vi "Force_2.vi"() -> ()   [LabVIEW 2020]
uses:
  Support/Controls/Cmd_Mouse Popup.ctl
  Support/Controls/Cmd_Var Data IO.ctl
  Support/Controls/Clst_Initialize Input.ctl
  Support/Controls/Clst_Result inspec.ctl
  Support/Public/Polymorph/Data Class_2D Str.vi
  Variables/Global_Cal Info.vi
  Support/Public/Polymorph/Rmv Empt Arr_2D Str.vi
panel:
  in  "Result set 2":string[][][](array[string])
  in  "Measured_ADJ":string[][](table) caption="● 측정 데이터 (조정후)"
  out "std set":string[][](table) caption="○ 분동 세트"
  in  "Spec Default set":string[][][](array[string])
  in  "Result set":string[][][](array[string])
  in  "CMC set":string[][][](array[string])
  in  "Resolution":string[][][](array[string])
  in  "condition 변경":bool
  in  "Spec set":string[][][](array[string])
  in  "Condition set":string[][][](array[string])
  in  "삭제":bool
  in  "단 선택":T1(ring)
  in  "dut info":i32(listbox) caption="교정대상 기기 정보"
  in  "Measured":string[][](table) caption="● 측정 데이터"
  in  "초기화":bool
  in  "적용":bool
  in  "지시형태":string(combo)="Digital"
  in  "교정범위":string(combo)="20 ~ 90 %"
  in  "사용 기준기":string(combo)
  in  "측정점 수":u8=5
  in  "단위":string(combo)="N"
  in  "최대 용량":dbl=10.0
  out "교정 방향":string="압축"
  in  "Spec 변경":bool
  in  "Random":bool
  out "Spec":string[][](table)
  out "제목":string
  out "에러 출력":errorcluster
  in  "최소눈금":dbl=0.001
  in  "Condition":string[][](table) caption="○ 상대지시 오차 교정"
  out "Load?":bool
  # "※ 교정하중 값을 변경하고 변경 적용 버튼을 클릭 !!"
  # "1차 (0˚)"
  # "2차 (120˚)"
  # "3차 (240˚)"
  # "1차 (0˚)"
  # "2차 (120˚)"
  # "3차 (240˚)"
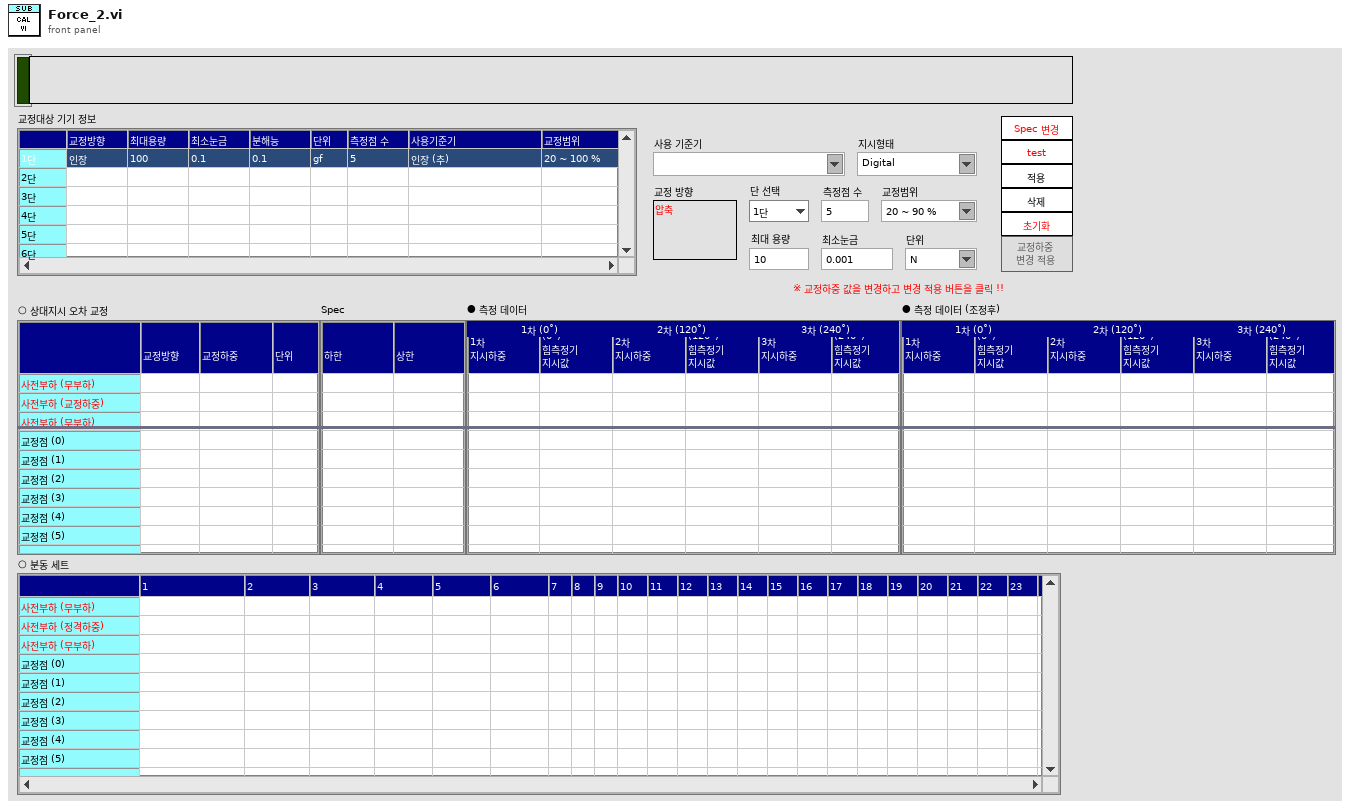
[diagram p1: front panel]
types:
  T1 = enum8{"1단", "2단", "3단", "4단", "5단", "6단", "7단", "8단", "9단", "10단"}
  T2 = typedef "Cmd_Mouse Popup.ctl" = enum16{"활성화", "메뉴선택"}
  T3 = typedef "Cmd_Var Data IO.ctl" = enum16{"Condition", "Condition Default", "Condition_Temp", "Resolution", "Resolution Default", "Resolution Old", "Spec", "Spec Default", "Spec Old", "Spec Temp", "Result", "Result2", "Result3", "Result_Temp", "Result_ADJ", "Result_ADJ2", "STD1", "STD2", "STD3", "STD4", "STD5", "STD Temp", "CMC", "CMC Default"}
  T4 = enum8{"Enabled", "Disabled", "Disabled and Grayed Out"}
  T5 = cluster{"Shift":bool, "Ctrl":bool, "Alt":bool, "Cmd":bool, "Opt":bool}
  T6 = typedef "Clst_Initialize Input.ctl" = cluster{"Initialize 1":cluster{"Condition":refnum<vi>[], "Spec":refnum<vi>[], "Measured":refnum<vi>[], "Resolution":refnum<vi>[], "Func_ext":string, "제목":refnum<vi>, "Measured_ADJ":refnum<vi>[]}, "Initialize 2":cluster{"문자열":refnum<vi>[], "콤보박스":refnum<vi>[], "링":refnum<vi>[], "열거형":refnum<vi>[], "테이블":refnum<vi>[], "여러열":refnum<vi>[], "디지털(DBL)":refnum<vi>[], "3D string":refnum<vi>[], "ctrl":refnum<vi>[], "boolean":refnum<vi>[]}}
  T7 = typedef "Clst_Result inspec.ctl" = cluster{"분해능":string, "문자열 1":string, "문자열 2":string, "숫자형 1":i32, "숫자형 2":i32, "숫자형 3":dbl, "문자배열 1D":string[], "문자배열 2D":string[][], "문자배열 3D":string[][][], "문자배열 4D":string[][][][], "불리언 1D":bool[]}
  T8 = cluster{"교정 방향":string, "최대 용량":dbl, "최소눈금":dbl, "지시형태":string, "단위":string, "측정점 수":u8, "사용 기준기":string, "사용 기준기 2":string, "단 선택":enum8{"1단", "2단", "3단", "4단", "5단", "6단", "7단", "8단", "9단", "10단"}, "ItemNames":string[][]}
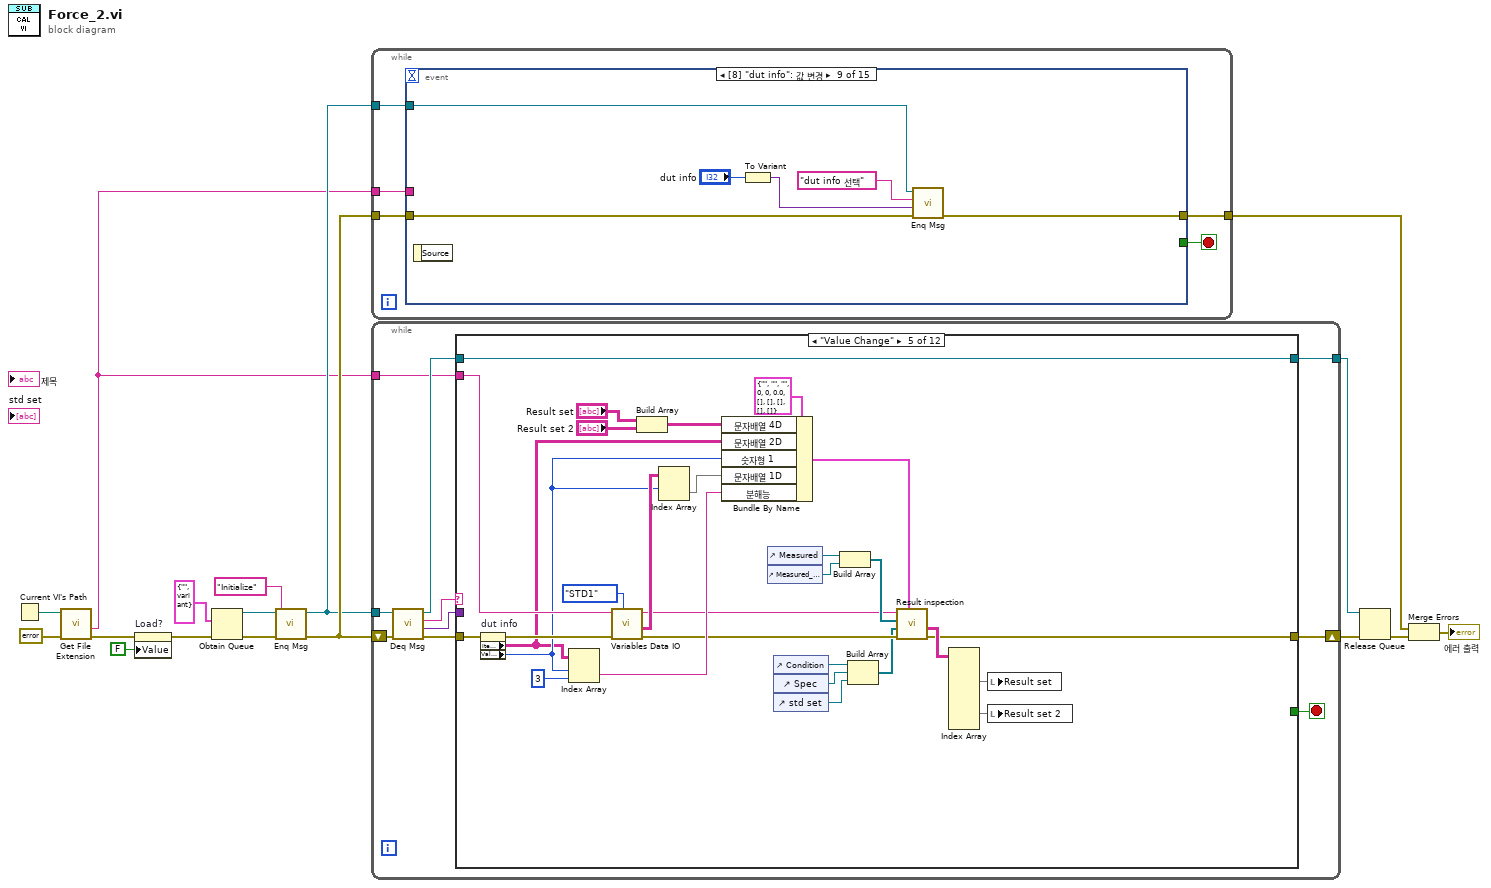
[diagram p0: block diagram]
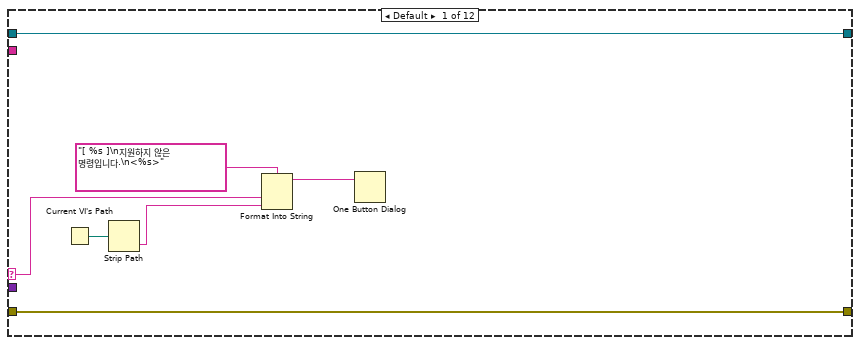
[diagram p2: hidden frame]
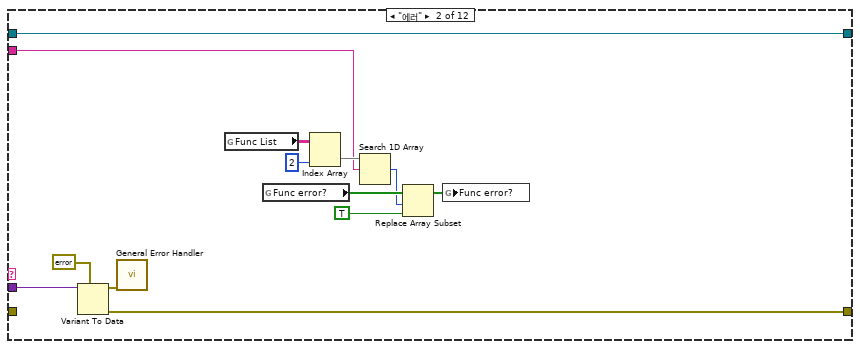
[diagram p3: hidden frame]
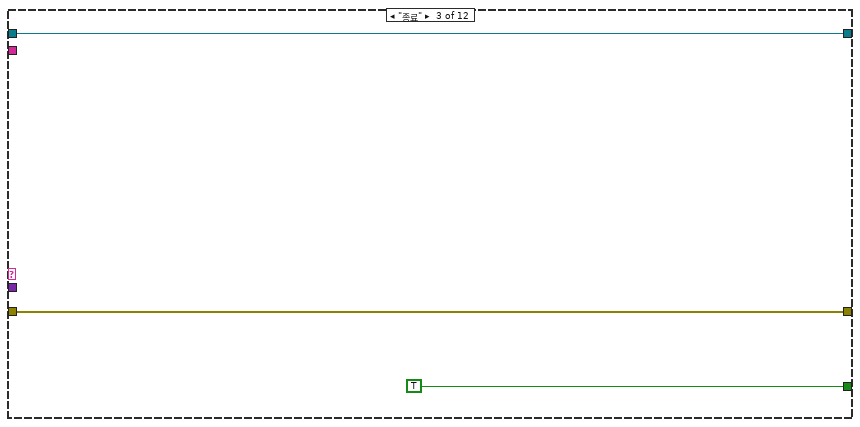
[diagram p4: hidden frame]
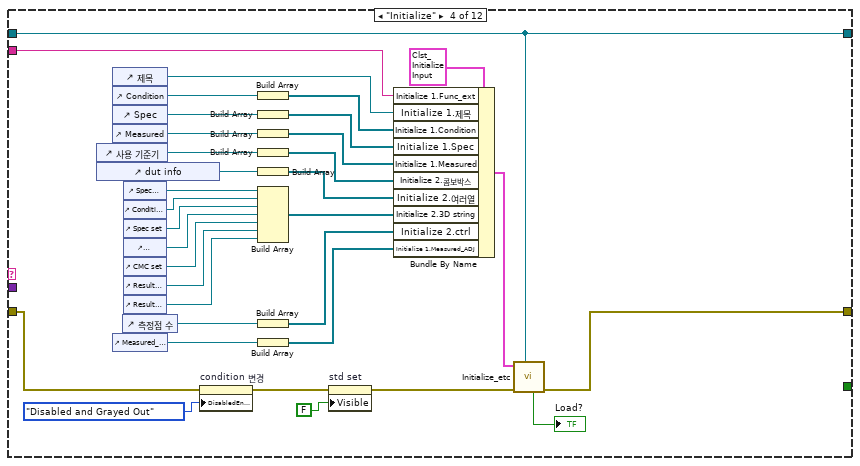
[diagram p5: hidden frame]
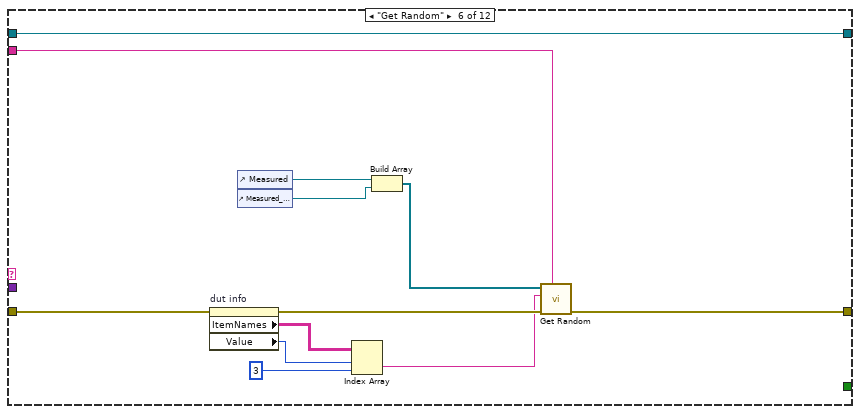
[diagram p6: hidden frame]
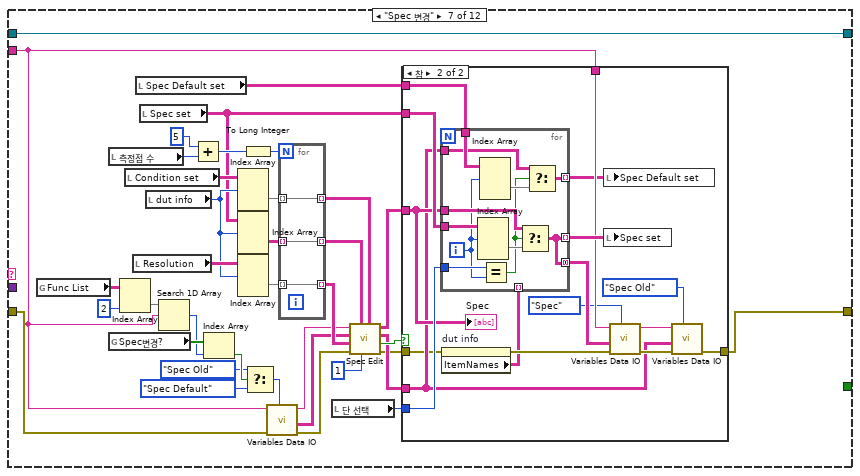
[diagram p7: hidden frame]
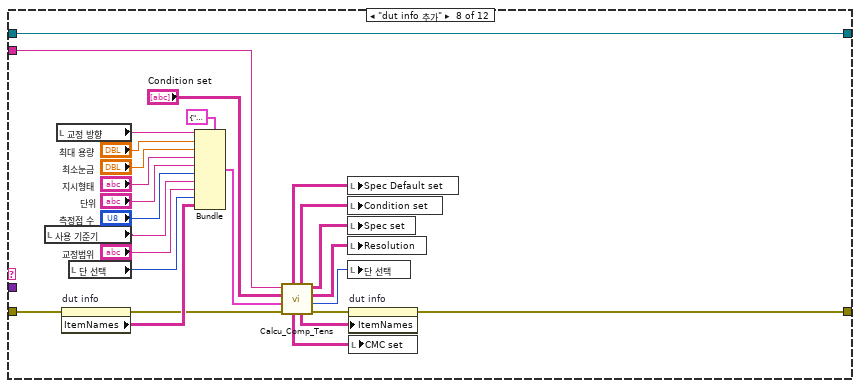
[diagram p9: hidden frame]
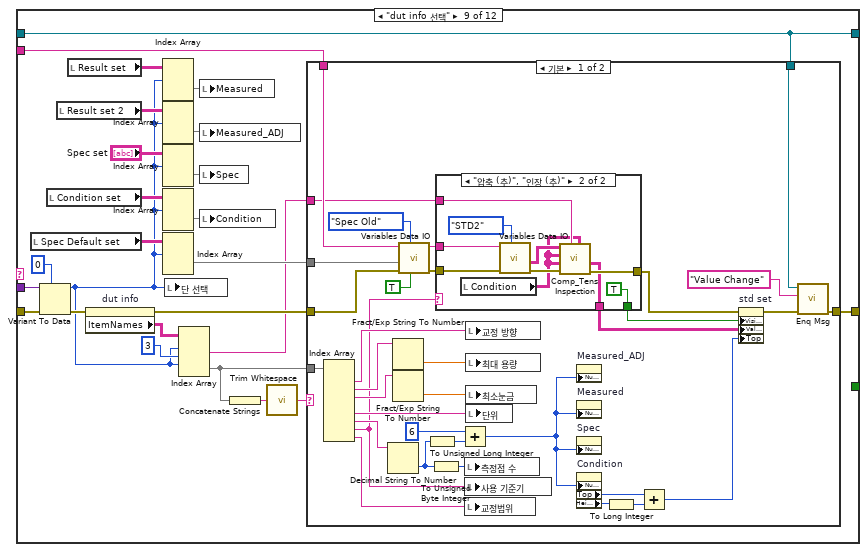
[diagram p10: hidden frame]
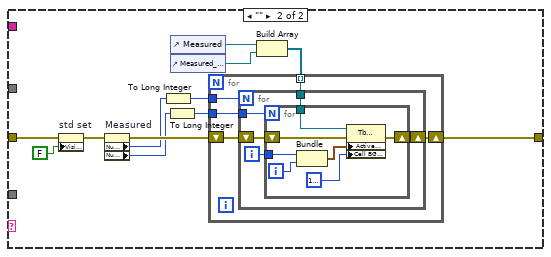
[diagram p12: hidden frame]
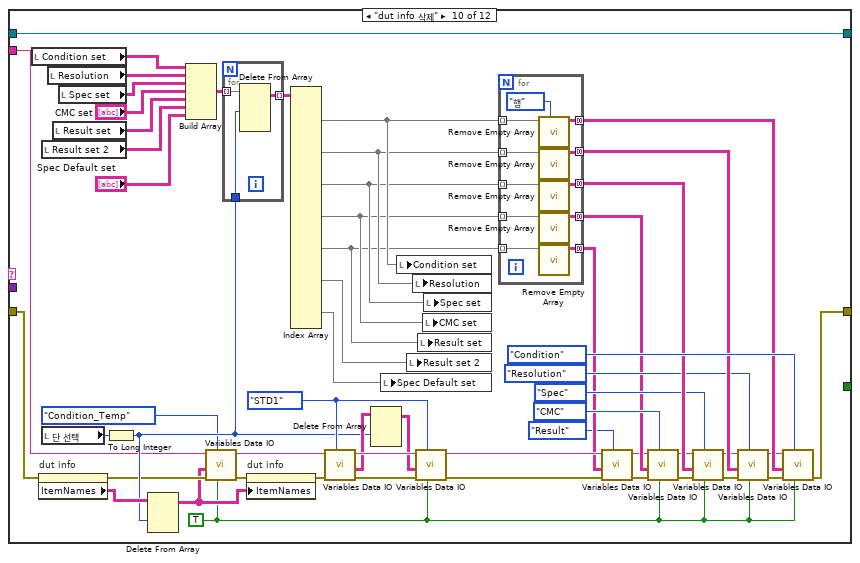
[diagram p13: hidden frame]
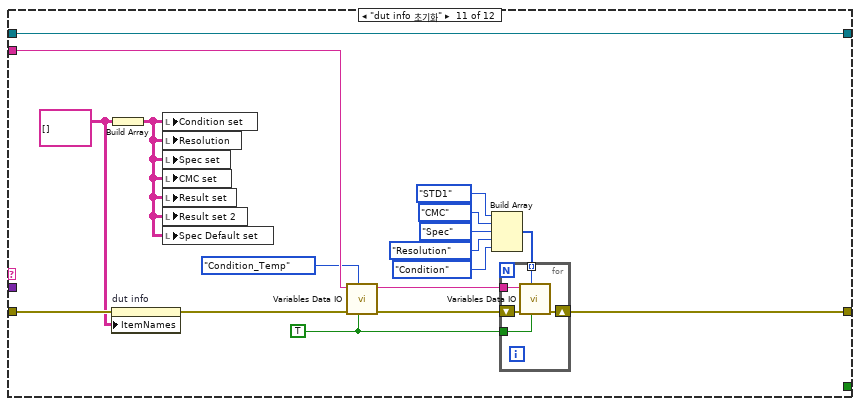
[diagram p14: hidden frame]
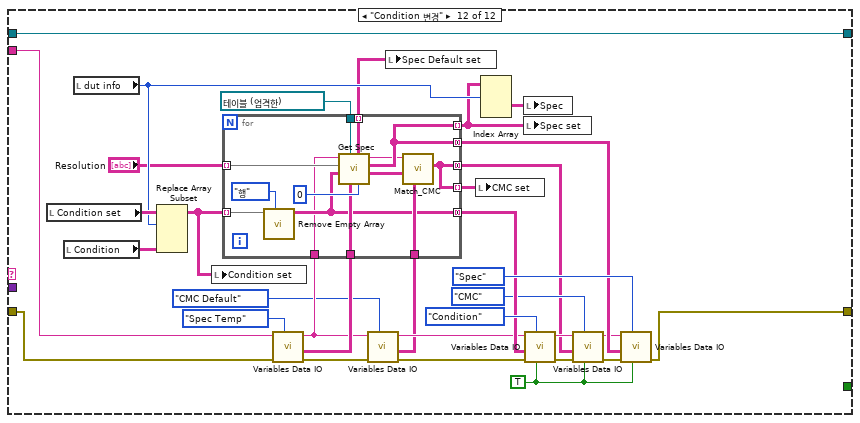
[diagram p15: hidden frame]
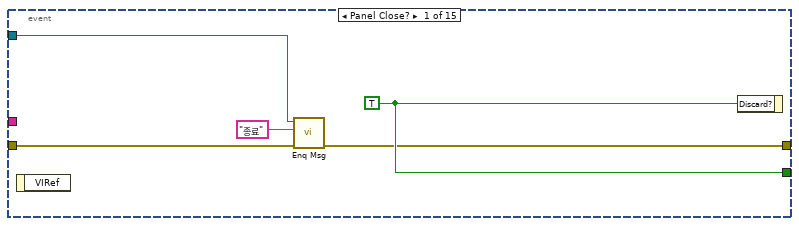
[diagram p16: hidden frame]
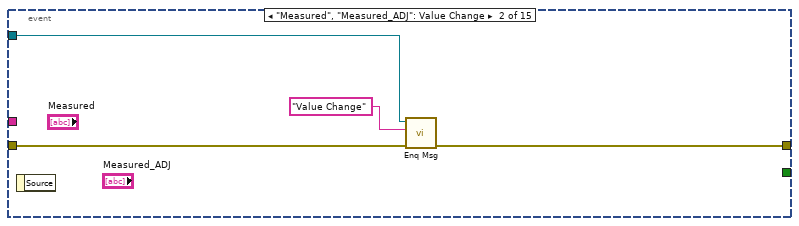
[diagram p17: hidden frame]
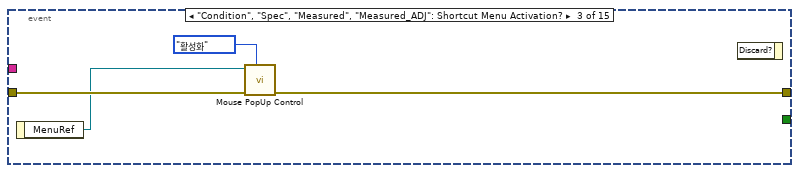
[diagram p18: hidden frame]
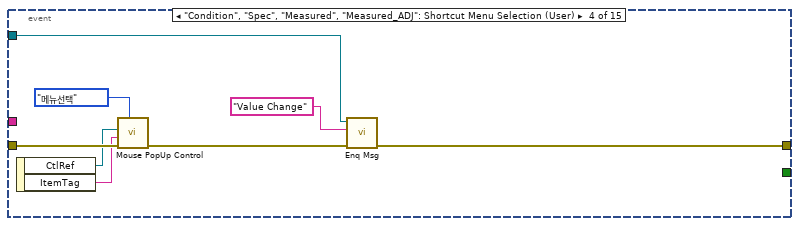
[diagram p19: hidden frame]
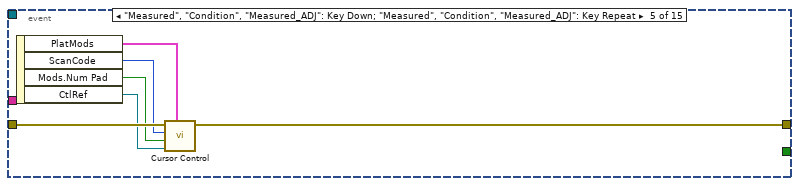
[diagram p20: hidden frame]
diagram:
  n1 = Current VI's Path() -> (path=w5:path)
  n2 = call <vilib>:"Get File Extension.vi"("error in (no error)"=errorcluster {"status"=FALSE, "code"=0, "source"=""} ("에러 상수"), "file"=w5) -> ("error out"=w3:errorcluster, "filename without extension"=w4:string)  [unwired: 5 in, 3 out]
  n3 = property on="Load?" class="Bool (엄격한)"(error in=w3, "Value"=FALSE ("Load?")) -> (error out=w2:errorcluster)  [unwired: 1 in, 1 out]
  n4 = Obtain Queue(element data type=cluster{"메세지":string, "값":variant} {"메세지"="", "값"=variant} ("Message Cluster"), error in (no error)=w2) -> (queue out=w14:refnum<queue>, error out=w16:errorcluster)  [unwired: 3 in, 1 out]
  n5 = call "Enq Msg.vi"("에러 입력(에러 없음)"=w16, "메세지"="Initialize", "큐 입력"=w14) -> ("에러 출력"=w15:errorcluster, "큐 출력"=w12:refnum<queue>)  [unwired: 7 in]
  n6 = while {
    tunnel: w15 -> [w20]
    tunnel: w12 -> [w21]
    tunnel: [w19] -> w9
    tunnel: w4 -> [w18]
    stop <- w22 stop-if-true
    n7 = event shown="[8] \"dut info\": 값 변경" {
      selector: _ -> [_ _ _ _ _ _ _ _ _ _ _ _ _ _ _]
      dyn-events: _ -> [_ _ _ _ _ _ _ _ _ _ _ _ _ _ _]
      timeout: _ -> [_ _ _ _ _ _ _ _ _ _ _ _ _ _ _]
      tunnel: [w27 _ _ _ _ _ _ _ _ _ _ _ _ _ _] -> w22
      tunnel: w21 -> [w25 w30 _ w37 _ w51 w57 w69 w76 w82 _ w99 w105 w132 _]
      tunnel: w20 -> [w26 w31 w34 w42 w49 w52 w59 w67 w73 w81 w95 w98 w104 w113 w152]
      tunnel: [w23 w28 w33 w36 w48 w50 w58 w70 w77 w83 w89 w100 w106 w133 w151] -> w19
      tunnel: w18 -> [_ _ _ _ _ _ _ _ _ _ w94 _ _ w120 _]
      event Panel Close? {
        w27 = TRUE ("버림?")
        n8 = event-data() -> ()  [unwired: 1 in, 1 out]
        n9 = call "Enq Msg.vi"("에러 입력(에러 없음)"=w26, "메세지"="종료", "큐 입력"=w25) -> ("에러 출력"=w23:errorcluster)  [unwired: 7 in, 1 out]
        n10 = event-data("Discard?"=w27) -> ()  [unwired: 1 in, 1 out]
      }
      event "Measured", "Measured_ADJ": Value Change {
        n11 = event-data() -> ()  [unwired: 1 in, 1 out]
        n12 = call "Enq Msg.vi"("에러 입력(에러 없음)"=w31, "메세지"="Value Change", "큐 입력"=w30) -> ("에러 출력"=w28:errorcluster)  [unwired: 7 in, 1 out]
      }
      event "Condition", "Spec", "Measured", "Measured_ADJ": Shortcut Menu Activation? {
        n13 = event-data() -> ("MenuRef"=w32:refnum<k9>)  [unwired: 1 in]
        n14 = call "Mouse PopUp Control.vi"("type"=Cmd_Mouse_Popup."활성화", "error in"=w34, "메뉴 참조"=w32) -> ("error out"=w33:errorcluster)  [unwired: 8 in]
        n15 = event-data() -> ()  [unwired: 2 in, 1 out]
      }
      event "Condition", "Spec", "Measured", "Measured_ADJ": Shortcut Menu Selection (User) {
        n16 = event-data() -> ("CtlRef"=w40:refnum<vi>, "ItemTag"=w41:string)  [unwired: 1 in]
        n17 = call "Mouse PopUp Control.vi"("type"=Cmd_Mouse_Popup."메뉴선택", "error in"=w42, "아이템 태그"=w41, "Tbl 참조 번호"=w40) -> ("error out"=w38:errorcluster)  [unwired: 7 in]
        n18 = call "Enq Msg.vi"("에러 입력(에러 없음)"=w38, "메세지"="Value Change", "큐 입력"=w37) -> ("에러 출력"=w36:errorcluster)  [unwired: 7 in, 1 out]
      }
      event "Measured", "Condition", "Measured_ADJ": Key Down; "Measured", "Condition", "Measured_ADJ": Key Repeat {
        n19 = event-data() -> ("PlatMods"=w44:T5, "ScanCode"=w47:i16, "Mods.Num Pad"=w46:bool, "CtlRef"=w45:refnum<vi>)  [unwired: 1 in]
        n20 = call "Cursor Control.vi"("플랫폼 조합키"=w44, "참조"=w45, "Num Pad"=w46, "ScanCode"=w47, "error in"=w49) -> ("error out"=w48:errorcluster)  [unwired: 5 in, 1 out]
      }
      event "Random": Value Change {
        n21 = event-data() -> ()  [unwired: 1 in, 1 out]
        n22 = call "Enq Msg.vi"("에러 입력(에러 없음)"=w52, "메세지"="Get Random", "큐 입력"=w51) -> ("에러 출력"=w54:errorcluster, "큐 출력"=w55:refnum<queue>)  [unwired: 7 in]
        n23 = call "Enq Msg.vi"("에러 입력(에러 없음)"=w54, "메세지"="Value Change", "큐 입력"=w55) -> ("에러 출력"=w50:errorcluster)  [unwired: 7 in, 1 out]
      }
      event "Spec 변경": Value Change {
        n24 = event-data() -> ()  [unwired: 1 in, 1 out]
        n25 = call "Enq Msg.vi"("에러 입력(에러 없음)"=w59, "메세지"="Spec 변경", "큐 입력"=w57) -> ("에러 출력"=w58:errorcluster)  [unwired: 7 in, 1 out]
      }
      event "적용": Value Change {
        w68 = string[][] []
        n26 = event-data() -> ()  [unwired: 1 in, 1 out]
        n27 = property on="dut info" class="MCListbox (엄격한)"(error in=w67, "Value"=-1 ("dut info")) -> (error out=w66:errorcluster, "ItemNames"=w65:string[][])  [unwired: 1 in, 1 out]
        n28 = Array Size(array=w65) -> (size(s)=w64:i32[])
        n29 = Index Array(array=w64) -> (element=w63:i32)  [unwired: 1 in]
        n30 = Equal To 0?(x=w63) -> (x = 0?=w62:bool)
        n31 = case shown="참" w62 {
          frame False {
          }
          frame True {
            n32 = local write "단 선택"(T1."1단" ("단 선택")) -> ()
          }
        }
        n33 = local write "Spec"(w68) -> ()
        n34 = local write "Condition"(w68) -> ()
        n35 = local write "Measured"(w68) -> ()
        n36 = call "Enq Msg.vi"("에러 입력(에러 없음)"=w66, "메세지"="dut info 추가", "큐 입력"=w69) -> ("에러 출력"=w70:errorcluster)  [unwired: 7 in, 1 out]
      }
      event "dut info": Value Change {
        n37 = event-data() -> ()  [unwired: 1 in, 1 out]
        n38 = To Variant(anything="dut info") -> (Variant=w74:variant)
        n39 = call "Enq Msg.vi"("에러 입력(에러 없음)"=w73, "값"=w74, "메세지"="dut info 선택", "큐 입력"=w76) -> ("에러 출력"=w77:errorcluster)  [unwired: 6 in, 1 out]
      }
      event "단 선택": Value Change {
        n40 = event-data() -> ()  [unwired: 1 in, 1 out]
        n41 = To Variant(anything="단 선택") -> (Variant=w80:variant)
        n42 = call "Enq Msg.vi"("에러 입력(에러 없음)"=w81, "값"=w80, "메세지"="dut info 선택", "큐 입력"=w82) -> ("에러 출력"=w83:errorcluster)  [unwired: 6 in, 1 out]
      }
      event "사용 기준기": Value Change {
        n43 = event-data() -> ()  [unwired: 1 in, 3 out]
        n44 = call "Variables Data IO.vi"("Select"=Cmd_Var_Data_IO."STD Temp", "error in"=w95, "Func_ext"=w94) -> ("error out"=w89:errorcluster, "Data Out"=w91:string[][])  [unwired: 6 in, 1 out]
        n45 = call-poly "Data Classification.vi"("인덱스"=6, "DATA 입력"=w91, "검색 문자열"="사용 기준기") -> ("DATA 출력"=w90:string[][])  [unwired: 4 in, 4 out]
        n46 = Index Array(array=w90, index (row)=0 ("인덱스 (행)"), index (col)=3 ("비활성화된 인덱스 (열)")) -> (element=→"교정 방향":string)
      }
      event "삭제": Value Change {
        w97 = string[][] []
        n47 = event-data() -> ()  [unwired: 1 in, 1 out]
        n48 = local write "dut info"(-1 ("dut info")) -> ()
        n49 = call "Enq Msg.vi"("에러 입력(에러 없음)"=w98, "메세지"="dut info 삭제", "큐 입력"=w99) -> ("에러 출력"=w100:errorcluster)  [unwired: 7 in, 1 out]
        n50 = local write "Spec"(w97) -> ()
        n51 = local write "Condition"(w97) -> ()
        n52 = local write "Measured"(w97) -> ()
      }
      event "초기화": Value Change {
        w103 = string[][] []
        n53 = event-data() -> ()  [unwired: 1 in, 1 out]
        n54 = local write "dut info"(-1 ("dut info")) -> ()
        n55 = call "Enq Msg.vi"("에러 입력(에러 없음)"=w104, "메세지"="dut info 초기화", "큐 입력"=w105) -> ("에러 출력"=w106:errorcluster)  [unwired: 7 in, 1 out]
        n56 = local write "Spec"(w103) -> ()
        n57 = local write "Condition"(w103) -> ()
        n58 = local write "Measured"(w103) -> ()
      }
      event "condition 변경": Value Change {
        n59 = event-data() -> ()  [unwired: 1 in, 1 out]
        n60 = property on="dut info" class="MCListbox (엄격한)"(error in=w113) -> (error out=w112:errorcluster, "ItemNames"=w111:string[][], "Value"=w110:i32)  [unwired: 1 in, 1 out]
        n61 = call "Variables Data IO.vi"("Select"=Cmd_Var_Data_IO."STD Temp", "error in"=w112, "Func_ext"=w120) -> ("error out"=w122:errorcluster, "Data Out"=w123:string[][])  [unwired: 6 in, 1 out]
        n62 = Index Array(array=w111, index (row)=w110, index (col)=6 ("비활성화된 인덱스 (열)")) -> (element=w108:string)
        n63 = local read "Condition"() -> (w118:string[][])
        n64 = call-poly "Data Classification.vi"("인덱스"=6, "DATA 입력"=w123, "검색 문자열"=w108) -> ("DATA 출력"=w130:string[][])  [unwired: 4 in, 4 out]
        n65 = Index Array(array=w130) -> (element=w125:string[])  [unwired: 2 in]
        n66 = Index Array(array=w118, index (col)=1 ("비활성화된 인덱스 (열)")) -> (element=w117:string[])  [unwired: 1 in]
        n67 = local read "단위"() -> (w119:string)
        n68 = Index Array(array=w125, index #1=4 ("인덱스")) -> (element #1=w128:string, element #2=w127:string)  [unwired: 1 in]
        n69 = Fract/Exp String To Number(string=w117) -> (number=w115:dbl[])  [unwired: 3 in, 1 out]
        n70 = call "Unit Conversion.vi"("환산단위"=w119, "입력단위"=w127, "입력값"=w128) -> ("환산값 (DBL)"=w126:dbl)  [unwired: 3 in, 5 out]
        n71 = Array Max & Min(array=w115) -> (max value=w114:dbl)  [unwired: 3 out]
        n72 = Greater Or Equal?(x=w126, y=w114) -> (x >= y?=w121:bool)
        n73 = case shown="참" w121 {
          tunnel: [w135 w145] -> w133
          tunnel: w132 -> [_ w144]
          tunnel: w122 -> [w135 w142]
          frame False {
            n74 = One Button Dialog(message="변경할 하중이 기준기 용량 보다 큼." ("메시지")) -> ()  [unwired: 1 in, 1 out]
          }
          frame True {
            n75 = property on="condition 변경" class="Bool"(error in=w142, "DisabledEnum"=T4."Disabled and Grayed Out" ("비활성화")) -> (error out=w141:errorcluster)  [unwired: 1 in, 1 out]
            n76 = control-ref of="Measured_ADJ"() -> (w137:refnum<vi>)
            n77 = Build Array(w137) -> (w136:refnum<vi>[])
            n78 = property on="Measured" class="Tbl (엄격한)"(error in=w141, "DisabledEnum"=T4."Enabled" ("비활성화")) -> (error out=w139:errorcluster)  [unwired: 1 in, 1 out]
            n79 = call "Meas_ADJ_Status.vi"("에러 입력(에러 없음)"=w139, "Measured_ADJ in"=w136) -> ("에러 출력"=w138:errorcluster)  [unwired: 8 in, 1 out]
            n80 = call "Enq Msg.vi"("에러 입력(에러 없음)"=w138, "메세지"="Condition 변경", "큐 입력"=w144) -> ("에러 출력"=w145:errorcluster)  [unwired: 7 in, 1 out]
          }
        }
      }
      event "Condition": Value Change {
        w147 = T4."Disabled and Grayed Out" ("비활성화")
        n81 = event-data() -> ()  [unwired: 1 in, 1 out]
        n82 = property on="Measured" class="Tbl (엄격한)"(error in=w152, "DisabledEnum"=w147) -> (error out=w149:errorcluster)  [unwired: 1 in, 1 out]
        n83 = property on="Measured_ADJ" class="Tbl (엄격한)"(error in=w149, "DisabledEnum"=w147) -> (error out=w148:errorcluster)  [unwired: 1 in, 1 out]
        n84 = property on="condition 변경" class="Bool"(error in=w148, "DisabledEnum"=T4."Enabled" ("비활성화")) -> (error out=w151:errorcluster)  [unwired: 1 in, 1 out]
      }
    }
  }
  n85 = while {
    shift-right: [w162] -> w11
    shift-left: w15 -> [w161]
    tunnel: w12 -> [w159]
    tunnel: [w154] -> w10
    tunnel: w4 -> [w153]
    stop <- w155 stop-if-true
    n86 = call "Deq Msg.vi"("에러 입력(에러 없음)"=w161, "큐 입력"=w159) -> ("에러 출력"=w160:errorcluster, "값"=w156:variant, "메세지"=w158:string, "큐 출력"=w157:refnum<queue>)  [unwired: 6 in]
    n87 = case shown="\"Value Change\"" w158 {
      selector: w158 -> [w165 _ _ _ _ _ _ _ _ _ _ _]
      tunnel: w160 -> [w169 _ w185 w200 w238 w255 w276 w354 w380 w508 w539 w576]
      tunnel: [w169 w179 w185 w209 w229 w258 w292 w345 w371 w504 w538 w573] -> w162
      tunnel: w157 -> [w168 w178 w183 w212 w248 w260 w297 w355 w361 w509 w540 w578]
      tunnel: w156 -> [_ w180 _ _ _ _ _ _ w379 _ _ _]
      tunnel: [_ _ TRUE ("버림?") _ _ _ _ _ _ _ _ _] -> w155
      tunnel: [w168 w178 w183 w212 w248 w260 w297 w355 w361 w509 w540 w578] -> w154
      tunnel: w153 -> [_ w170 _ w208 w243 w256 w263 w333 w365 w464 w529 w574]
      frame Default {
        n88 = Current VI's Path() -> (path=w164:path)
        n89 = Strip Path(path=w164) -> (name=w163:string)  [unwired: 1 out]
        n90 = Format Into String(format string="[ %s ]\n지원하지 않은 명령입니다.\n<%s>" ("메시지"), w165, w163) -> (resulting string=w166:string)  [unwired: 2 in, 1 out]
        n91 = One Button Dialog(message=w166) -> ()  [unwired: 1 in, 1 out]
      }
      frame "에러" {
        n92 = Variant To Data(type=errorcluster {"status"=FALSE, "code"=0, "source"=""} ("에러 출력"), Variant=w180) -> (data=w182:errorcluster, error out=w179:errorcluster)  [unwired: 1 in]
        n93 = call <vilib>:"General Error Handler.vi"("error in (no error)"=w182) -> ()  [unwired: 10 in, 5 out]
        n94 = global read "Global_Cal Info.vi" "Func List"() -> (w176:string[][])
        n95 = global read "Global_Cal Info.vi" "Func error?"() -> (w173:bool[])
        n96 = Index Array(array=w176, index (col)=2 ("비활성화된 인덱스 (열)")) -> (element=w175:string[])  [unwired: 1 in]
        n97 = Search 1D Array(1D array=w175, element=w170) -> (index of element=w172:i32)  [unwired: 1 in]
        n98 = Replace Array Subset(array=w173, new element=TRUE ("새 원소/부분배열"), index=w172) -> (w171:bool[])
        n99 = global write "Global_Cal Info.vi" "Func error?"(w171) -> ()
      }
      frame "종료" {
      }
      frame "Initialize" {
        n100 = control-ref of="사용 기준기"() -> (w207:refnum<vi>)
        n101 = control-ref of="dut info"() -> (w204:refnum<vi>)
        n102 = control-ref of="제목"() -> (w214:refnum<vi>)
        n103 = control-ref of="Condition"() -> (w211:refnum<vi>)
        n104 = control-ref of="Spec"() -> (w210:refnum<vi>)
        n105 = control-ref of="Measured"() -> (w215:refnum<vi>)
        n106 = control-ref of="Measured_ADJ"() -> (w190:refnum<vi>)
        n107 = control-ref of="측정점 수"() -> (w199:refnum<vi>)
        n108 = control-ref of="Spec Default set"() -> (w203:refnum<vi>)
        n109 = control-ref of="Condition set"() -> (w197:refnum<vi>)
        n110 = control-ref of="Spec set"() -> (w196:refnum<vi>)
        n111 = control-ref of="Resolution"() -> (w195:refnum<vi>)
        n112 = control-ref of="CMC set"() -> (w194:refnum<vi>)
        n113 = control-ref of="Result set"() -> (w188:refnum<vi>)
        n114 = control-ref of="Result set 2"() -> (w187:refnum<vi>)
        n115 = property on="condition 변경" class="Bool"(error in=w200, "DisabledEnum"=T4."Disabled and Grayed Out" ("비활성화")) -> (error out=w193:errorcluster)  [unwired: 1 in, 1 out]
        n116 = Build Array(w211) -> (w217:refnum<vi>[])
        n117 = Build Array(w210) -> (w213:refnum<vi>[])
        n118 = Build Array(w215) -> (w216:refnum<vi>[])
        n119 = Build Array(w207) -> (w206:refnum<vi>[])
        n120 = Build Array(w204) -> (w205:refnum<vi>[])
        n121 = Build Array(w203, w197, w196, w195, w194, w188, w187) -> (w202:refnum<vi>[])
        n122 = Build Array(w199) -> (w198:refnum<vi>[])
        n123 = Build Array(w190) -> (w189:refnum<vi>[])
        n124 = property on="std set" class="Tbl (엄격한)"(error in=w193, "Visible"=FALSE ("보이기")) -> (error out=w192:errorcluster)  [unwired: 1 in, 1 out]
        n125 = Bundle By Name(cluster=T6 {"Initialize 1"={"Condition"=[], "Spec"=[], "Measured"=[], "Resolution"=[], "Func_ext"="", "제목"=refnum, "Measured_ADJ"=[]}, "Initialize 2"={"문자열"=[], "콤보박스"=[], "링"=[], "열거형"=[], "테이블"=[], "여러열"=[], "디지털(DBL)"=[], "3D string"=[], "ctrl"=[], "boolean"=[]}} ("입력 클러스터"), "Initialize 1.Func_ext"=w208, "Initialize 1.제목"=w214, "Initialize 1.Condition"=w217, "Initialize 1.Spec"=w213, "Initialize 1.Measured"=w216, "Initialize 2.콤보박스"=w206, "Initialize 2.여러열"=w205, "Initialize 2.3D string"=w202, "Initialize 2.ctrl"=w198, "Initialize 1.Measured_ADJ"=w189) -> (w218:T6)
        n126 = call "Initialize_etc.vi"("큐 입력"=w212, "error in"=w192, "입력 클러스터"=w218) -> ("error out"=w209:errorcluster, "Load?"=→"Load?":bool)  [unwired: 6 in, 1 out]
      }
      frame "Value Change" {
        n127 = property on="dut info" class="MCListbox (엄격한)"(error in=w238) -> (error out=w237:errorcluster, "ItemNames"=w233:string[][], "Value"=w234:i32)  [unwired: 1 in, 1 out]
        n128 = Index Array(array=w233, index (row)=w234, index (col)=3 ("비활성화된 인덱스 (열)")) -> (element=w239:string)
        n129 = call "Variables Data IO.vi"("Select"=Cmd_Var_Data_IO."STD1", "error in"=w237, "Func_ext"=w243) -> ("error out"=w236:errorcluster, "Data Out"=w241:string[][], "Func_ext Out"=w228:string)  [unwired: 6 in]
        n130 = Build Array("Result set", "Result set 2") -> (w224:string[][][][])
        n131 = Index Array(array=w241, index (row)=w234) -> (element=w235:string[])  [unwired: 1 in]
        n132 = Bundle By Name(cluster=T7 {"분해능"="", "문자열 1"="", "문자열 2"="", "숫자형 1"=0, "숫자형 2"=0, "숫자형 3"=0.0, "문자배열 1D"=[], "문자배열 2D"=[], "문자배열 3D"=[], "문자배열 4D"=[], "불리언 1D"=[]} ("입력 클러스터"), "문자배열 4D"=w224, "문자배열 2D"=w233, "숫자형 1"=w234, "문자배열 1D"=w235, "분해능"=w239) -> (w225:T7)
        n133 = control-ref of="Measured"() -> (w227:refnum<vi>)
        n134 = control-ref of="Measured_ADJ"() -> (w222:refnum<vi>)
        n135 = control-ref of="Condition"() -> (w245:refnum<vi>)
        n136 = control-ref of="Spec"() -> (w244:refnum<vi>)
        n137 = control-ref of="std set"() -> (w231:refnum<vi>)
        n138 = Build Array(w227, w222) -> (w247:refnum<vi>[])
        n139 = Build Array(w245, w244, w231) -> (w226:refnum<vi>[])
        n140 = call "Result inspection.vi"("입력 클러스터"=w225, "error in"=w236, "Ref. Data (excluded)"=w226, "Ref. Data (Inspection)"=w247, "Func ext"=w228) -> ("error out"=w229:errorcluster, "Data 3D"=w230:string[][][][])  [unwired: 3 in, 2 out]
        n141 = Index Array(array=w230) -> (element #1=w221:string[][][], element #2=w220:string[][][])  [unwired: 8 in]
        n142 = local write "Result set"(w221) -> ()
        n143 = local write "Result set 2"(w220) -> ()
      }
      frame "Get Random" {
        n144 = property on="dut info" class="MCListbox (엄격한)"(error in=w255) -> (error out=w254:errorcluster, "ItemNames"=w253:string[][], "Value"=w251:i32)  [unwired: 1 in, 1 out]
        n145 = control-ref of="Measured"() -> (w257:refnum<vi>)
        n146 = control-ref of="Measured_ADJ"() -> (w249:refnum<vi>)
        n147 = Index Array(array=w253, index (row)=w251, index (col)=3 ("비활성화된 인덱스 (열)")) -> (element=w250:string)
        n148 = Build Array(w257, w249) -> (w259:refnum<vi>[])
        n149 = call "Get Random.vi"("Func_Ext"=w256, "에러 입력"=w254, "분해능"=w250, "Meas"=w259) -> ("에러 출력"=w258:errorcluster)  [unwired: 6 in, 1 out]
      }
      frame "Spec 변경" {
        n150 = global read "Global_Cal Info.vi" "Func List"() -> (w270:string[][])
        n151 = local read "측정점 수"() -> (w282:u8)
        n152 = global read "Global_Cal Info.vi" "Spec변경?"() -> (w274:bool[])
        n153 = Index Array(array=w270, index (col)=2 ("비활성화된 인덱스 (열)")) -> (element=w272:string[])  [unwired: 1 in]
        n154 = local read "Condition set"() -> (w291:string[][][])
        n155 = local read "Resolution"() -> (w290:string[][][])
        n156 = local read "Spec Default set"() -> (w261:string[][][])
        n157 = local read "Spec set"() -> (w278:string[][][])
        n158 = local read "dut info"() -> (w289:i32)
        n159 = Search 1D Array(1D array=w272, element=w263) -> (index of element=w273:i32)  [unwired: 1 in]
        n160 = Add(x=u8 5, y=w282) -> (x+y=w280:u8)
        n161 = Index Array(array=w274, index=w273) -> (element=w269:bool)
        n162 = Index Array(array=w291, index (dim 0)=w289) -> (element=w288:string[][])  [unwired: 2 in]
        n163 = Index Array(array=w278, index (dim 0)=w289) -> (element=w287:string[][])  [unwired: 2 in]
        n164 = Index Array(array=w290, index (dim 0)=w289) -> (element=w286:string[][])  [unwired: 2 in]
        n165 = To Long Integer(number=w280) -> (32bit integer=w281:i32)
        n166 = Select(t=Cmd_Var_Data_IO."Spec Old" ("Select"), s=w269, f=Cmd_Var_Data_IO."Spec Default" ("Select")) -> (s? t:f=w266:T3)
        n167 = call "Variables Data IO.vi"("Select"=w266, "error in"=w276, "Func_ext"=w263) -> ("error out"=w275:errorcluster, "Data Out"=w262:string[][], "Func_ext Out"=w265:string)  [unwired: 6 in]
        n168 = for {
          N: w281 -> [_]
          tunnel: w288 -> [w298] mode=indexing
          tunnel: w287 -> [w299] mode=indexing
          tunnel: w286 -> [w300] mode=indexing
          tunnel: [w300] -> w285 mode=indexing
          tunnel: [w299] -> w284 mode=indexing
          tunnel: [w298] -> w283 mode=indexing
        }
        n169 = local read "단 선택"() -> (w277:T1)
        n170 = call "Spec Edit.vi"("Condition"=w283, "열번호(기준값)"=1 ("기준열(0)"), "Spec Value"=w284, "에러 입력(에러 없음)"=w275, "Resolution"=w285, "Spec Default"=w262, "Func_ext"=w265) -> ("에러 출력"=w294:errorcluster, "변경?"=w296:bool, "Spec Default out"=w295:string[][], "Spec 출력"=w264:string[][])  [unwired: 1 in]
        n171 = case shown="참" w296 {
          tunnel: w294 -> [w301 w304]
          tunnel: [w301 w309] -> w292
          tunnel: w264 -> [_ w312]
          tunnel: w263 -> [_ w316]
          tunnel: w295 -> [_ w306]
          tunnel: w278 -> [_ w318]
          tunnel: w277 -> [_ w313]
          tunnel: w261 -> [_ w307]
          frame False {
          }
          frame True {
            n172 = property on="dut info" class="MCListbox (엄격한)"(error in=w304) -> (error out=w303:errorcluster, "ItemNames"=w302:string[][])  [unwired: 1 in, 1 out]
            n173 = for {
              tunnel: w318 -> [w328]
              tunnel: [w323] -> w317 mode=indexing
              tunnel: w313 -> [w326]
              tunnel: w312 -> [w329]
              tunnel: [w323] -> w315 mode=concatenating
              tunnel: w307 -> [w325]
              tunnel: w306 -> [w321]
              tunnel: [w320] -> w305 mode=indexing
              tunnel: w302 -> [_] mode=indexing
              i -> [w324]
              n174 = Index Array(array=w328, index (dim 0)=w324) -> (element=w327:string[][])  [unwired: 2 in]
              n175 = Index Array(array=w325, index (dim 0)=w324) -> (element=w322:string[][])  [unwired: 2 in]
              n176 = Equal?(x=w326, y=w324) -> (x = y?=w319:bool)
              n177 = Select(t=w329, s=w319, f=w327) -> (s? t:f=w323:string[][])
              n178 = Select(t=w321, s=w319, f=w322) -> (s? t:f=w320:string[][])
            }
            n179 = local write "Spec Default set"(w305) -> ()
            n180 = local write "Spec set"(w317) -> ()
            n181 = call "Variables Data IO.vi"("Select"=Cmd_Var_Data_IO."Spec", "error in"=w303, "Data In"=w315, "Func_ext"=w316) -> ("error out"=w311:errorcluster, "Func_ext Out"=w310:string)  [unwired: 5 in, 1 out]
            n182 = call "Variables Data IO.vi"("Select"=Cmd_Var_Data_IO."Spec Old", "error in"=w311, "Data In"=w306, "Func_ext"=w310) -> ("error out"=w309:errorcluster)  [unwired: 5 in, 2 out]
            "Spec" <- w312
          }
        }
      }
      frame "dut info 추가" {
        n183 = local read "사용 기준기"() -> (w331:string)
        n184 = local read "교정 방향"() -> (w330:string)
        n185 = property on="dut info" class="MCListbox (엄격한)"(error in=w354) -> (error out=w344:errorcluster, "ItemNames"=w347:string[][])  [unwired: 1 in, 1 out]
        n186 = local read "단 선택"() -> (w342:T1)
        n187 = Bundle(cluster=T8 {"교정 방향"="", "최대 용량"=0.0, "최소눈금"=0.0, "지시형태"="", "단위"="", "측정점 수"=0, "사용 기준기"="", "사용 기준기 2"="", "단 선택"=enum."1단", "ItemNames"=[]} ("클러스터"), "교정 방향"=w330, "최대 용량"="최대 용량", "최소눈금"="최소눈금", "지시형태"="지시형태", "단위"="단위", "측정점 수"="측정점 수", "사용 기준기"=w331, "사용 기준기 2"="교정범위", "단 선택"=w342, "ItemNames"=w347) -> (w335:T8)
        n188 = call "Calcu_Comp_Tens.vi"("error in"=w344, "클러스터"=w335, "Condition set"="Condition set", "Func_ext"=w333) -> ("error out"=w343:errorcluster, "단 번호"=w338:i32, "Resolution"=w337:string[][][], "Spec Out"=w340:string[][][], "ItemNames 출력"=w339:string[][], "condition out"=w341:string[][][], "cmc out"=w336:string[][][], "Spec Default"=w332:string[][][])
        n189 = local write "Spec Default set"(w332) -> ()
        n190 = local write "Condition set"(w341) -> ()
        n191 = local write "Spec set"(w340) -> ()
        n192 = local write "Resolution"(w337) -> ()
        n193 = local write "단 선택"(w338) -> ()
        n194 = property on="dut info" class="MCListbox (엄격한)"(error in=w343, "ItemNames"=w339) -> (error out=w345:errorcluster)  [unwired: 1 in, 1 out]
        n195 = local write "CMC set"(w336) -> ()
      }
      frame "dut info 선택" {
        n196 = local read "Spec Default set"() -> (w367:string[][][])
        n197 = Variant To Data(error in=w380, type=0, Variant=w379) -> (data=w357:i32, error out=w375:errorcluster)
        n198 = local read "Condition set"() -> (w377:string[][][])
        n199 = local read "Result set 2"() -> (w359:string[][][])
        n200 = local read "Result set"() -> (w369:string[][][])
        n201 = property on="dut info" class="MCListbox (엄격한)"(error in=w375) -> (error out=w372:errorcluster, "ItemNames"=w374:string[][])  [unwired: 1 in, 1 out]
        n202 = Index Array(array=w369, index (dim 0)=w357) -> (element=w368:string[][])  [unwired: 2 in]
        n203 = Index Array(array=w359, index (dim 0)=w357) -> (element=w360:string[][])  [unwired: 2 in]
        n204 = Index Array(array="Spec set", index (dim 0)=w357) -> (element=w373:string[][])  [unwired: 2 in]
        n205 = Index Array(array=w377, index (dim 0)=w357) -> (element=w376:string[][])  [unwired: 2 in]
        n206 = Index Array(array=w367, index (dim 0)=w357) -> (element=w366:string[][])  [unwired: 2 in]
        n207 = local write "단 선택"(w357) -> ()
        n208 = Index Array(array=w374, index (row) #1=w357, index (col) #1=3 ("비활성화된 인덱스 (열)"), index (row) #2=w357) -> (element #1=w356:string, element #2=w364:string[])  [unwired: 1 in]
        n209 = local write "Measured"(w368) -> ()
        n210 = local write "Measured_ADJ"(w360) -> ()
        n211 = local write "Spec"(w373) -> ()
        n212 = local write "Condition"(w376) -> ()
        n213 = Concatenate Strings(w364) -> (w363:string)
        n214 = call <vilib>:"Trim Whitespace.vi"("string"=w363) -> ("trimmed string"=w362:string)  [unwired: 1 in]
        n215 = case shown="기본" w362 {
          tunnel: w364 -> [w414 _]
          tunnel: w372 -> [w402 w431]
          tunnel: [w396 w436] -> w371
          tunnel: w366 -> [w401 _]
          tunnel: w365 -> [w400 _]
          tunnel: w361 -> [w395 _]
          tunnel: w356 -> [w382 _]
          frame Default {
            n216 = Index Array(array=w414) -> (element #1=w413:string, element #2=w412:string, element #3=w409:string, element #5=w408:string, element #6=w407:string, element #7=w390:string, element #8=w406:string)  [unwired: 8 in, 1 out]
            n217 = Decimal String To Number(string=w407) -> (number=w384:i32)  [unwired: 2 in, 1 out]
            n218 = Fract/Exp String To Number(string=w412) -> (number=w411:dbl)  [unwired: 3 in, 1 out]
            n219 = Fract/Exp String To Number(string=w409) -> (number=w410:dbl)  [unwired: 3 in, 1 out]
            n220 = call "Variables Data IO.vi"("Write blank data ?(F)"=TRUE ("Write blank data ?(T)"), "Select"=Cmd_Var_Data_IO."Spec Old", "error in"=w402, "Data In"=w401, "Func_ext"=w400) -> ("error out"=w385:errorcluster, "Func_ext Out"=w386:string)  [unwired: 4 in, 1 out]
            n221 = To Unsigned Long Integer(number=w384) -> (unsigned 32bit integer=w383:u32)
            n222 = To Unsigned Byte Integer(number=w384) -> (unsigned 8bit integer=w405:u8)
            n223 = case shown="\"압축 (추)\", \"인장 (추)\"" w390 {
              tunnel: [_ TRUE] -> w389
              tunnel: [w415 w424] -> w387
              tunnel: w385 -> [w415 w423]
              tunnel: w386 -> [_ w420]
              tunnel: w382 -> [_ w418]
              tunnel: [_ w417] -> w381
              frame Default {
              }
              frame "압축 (추)", "인장 (추)" {
                n224 = local read "Condition"() -> (w416:string[][])
                n225 = call "Variables Data IO.vi"("Select"=Cmd_Var_Data_IO."STD2", "error in"=w423, "Func_ext"=w420) -> ("error out"=w422:errorcluster, "Data Out"=w421:string[][])  [unwired: 6 in, 1 out]
                n226 = call "Comp_Tens Inspection.vi"("Value"=w416, "분해능"=w418, "error in (no error)"=w422, "Spec"=w416, "Condition"=w416, "STD"=w421) -> ("error out"=w424:errorcluster, "사용기준추"=w417:string[][])  [unwired: 2 in, 2 out]
              }
            }
            n227 = Add(x=u32 6 ("y"), y=w383) -> (x+y=w403:u32)
            n228 = local write "측정점 수"(w405) -> ()
            n229 = local write "사용 기준기"(w390) -> ()
            n230 = local write "교정범위"(w406) -> ()
            n231 = local write "교정 방향"(w413) -> ()
            n232 = local write "최대 용량"(w411) -> ()
            n233 = local write "최소눈금"(w410) -> ()
            n234 = local write "단위"(w408) -> ()
            n235 = property on="Measured_ADJ" class="Tbl (엄격한)"("Number of Rows"=w403) -> ()  [unwired: 2 in, 2 out]
            n236 = property on="Measured" class="Tbl (엄격한)"("Number of Rows"=w403) -> ()  [unwired: 2 in, 2 out]
            n237 = property on="Spec" class="Tbl (엄격한)"("Number of Rows"=w403) -> ()  [unwired: 2 in, 2 out]
            n238 = property on="Condition" class="Tbl (엄격한)"("Number of Rows"=w403) -> ("Top"=w394:i32, "Height"=w393:u32)  [unwired: 2 in, 2 out]
            n239 = To Long Integer(number=w393) -> (32bit integer=w391:i32)
            n240 = Add(x=w394, y=w391) -> (x+y=w392:i32)
            n241 = property on="std set" class="Tbl (엄격한)"(error in=w387, "Visible"=w389, "Value"=w381, "Top"=w392) -> (error out=w388:errorcluster)  [unwired: 1 in, 1 out]
            n242 = call "Enq Msg.vi"("에러 입력(에러 없음)"=w388, "메세지"="Value Change", "큐 입력"=w395) -> ("에러 출력"=w396:errorcluster)  [unwired: 7 in, 1 out]
          }
          frame "" {
            n243 = property on="std set" class="Tbl (엄격한)"(error in=w431, "Visible"=FALSE ("보이기")) -> (error out=w430:errorcluster)  [unwired: 1 in, 1 out]
            n244 = property on="Measured" class="Tbl (엄격한)"(error in=w430) -> (error out=w437:errorcluster, "Number of Rows"=w435:u32, "Number of Columns"=w434:u32)  [unwired: 1 in, 1 out]
            n245 = To Long Integer(number=w435) -> (32bit integer=w433:i32)
            n246 = To Long Integer(number=w434) -> (32bit integer=w432:i32)
            n247 = control-ref of="Measured"() -> (w428:refnum<vi>)
            n248 = control-ref of="Measured_ADJ"() -> (w427:refnum<vi>)
            n249 = Build Array(w428, w427) -> (w426:refnum<vi>[])
            n250 = for {
              tunnel: w433 -> [w440]
              tunnel: w432 -> [w439]
              shift-right: [w441] -> w436
              shift-left: w437 -> [w442]
              tunnel: w426 -> [w438] mode=indexing
              n251 = for {
                N: w440 -> [_]
                shift-right: [w446] -> w441
                shift-left: w442 -> [w447]
                tunnel: w439 -> [w445]
                tunnel: w438 -> [w443]
                i -> [w444]
                n252 = for {
                  N: w445 -> [_]
                  shift-right: [w450] -> w446
                  shift-left: w447 -> [w451]
                  tunnel: w444 -> [w454]
                  tunnel: w443 -> [w448]
                  i -> [w453]
                  n253 = Bundle(w454, w453) -> (w452:cluster{i32, i32})  [unwired: 1 in]
                  n254 = property on="프로퍼티 노드" class="Tbl (엄격한)"(reference=w448, error in=w451, "Active Cell"=w452, "Cell BG Color"=u32 16777226) -> (error out=w450:errorcluster)  [unwired: 1 out]
                }
              }
            }
          }
        }
      }
      frame "dut info 삭제" {
        w459 = TRUE ("Write blank data ?(T)")
        w499 = Cmd_Var_Data_IO."STD1" ("Select")
        n255 = local read "Condition set"() -> (w496:string[][][])
        n256 = property on="dut info" class="MCListbox (엄격한)"(error in=w508) -> (error out=w465:errorcluster, "ItemNames"=w507:string[][])  [unwired: 1 in, 1 out]
        n257 = local read "Result set 2"() -> (w457:string[][][])
        n258 = local read "단 선택"() -> (w506:T1)
        n259 = local read "Resolution"() -> (w495:string[][][])
        n260 = local read "Result set"() -> (w473:string[][][])
        n261 = local read "Spec set"() -> (w494:string[][][])
        n262 = To Long Integer(number=w506) -> (32bit integer=w492:i32)
        n263 = Delete From Array(array=w507, index (row)=w492) -> (array with subset deleted=w461:string[][])  [unwired: 2 in, 1 out]
        n264 = Build Array(w496, w495, w494, "CMC set", w473, w457, "Spec Default set") -> (w493:string[][][][])
        n265 = call "Variables Data IO.vi"("Write blank data ?(F)"=w459, "Select"=Cmd_Var_Data_IO."Condition_Temp", "error in"=w465, "Data In"=w461, "Func_ext"=w464) -> ("error out"=w462:errorcluster, "Func_ext Out"=w463:string)  [unwired: 4 in, 1 out]
        n266 = for {
          tunnel: w493 -> [w512] mode=indexing
          tunnel: w492 -> [w511]
          tunnel: [w510] -> w491 mode=indexing
          n267 = Delete From Array(array=w512, index (dim 0)=w511) -> (array with subset deleted=w510:string[][][])  [unwired: 3 in, 1 out]
        }
        n268 = property on="dut info" class="MCListbox (엄격한)"(error in=w462, "ItemNames"=w461) -> (error out=w502:errorcluster)  [unwired: 1 in, 1 out]
        n269 = Index Array(array=w491) -> (element #1=w490:string[][][], element #2=w489:string[][][], element #3=w488:string[][][], element #4=w479:string[][][], element #5=w472:string[][][], element #6=w455:string[][][], element #7=w456:string[][][])  [unwired: 28 in]
        n270 = call "Variables Data IO.vi"("Select"=w499, "error in"=w502, "Func_ext"=w463) -> ("error out"=w500:errorcluster, "Data Out"=w498:string[][], "Func_ext Out"=w501:string)  [unwired: 6 in]
        n271 = Delete From Array(array=w498, index (row)=w492) -> (array with subset deleted=w497:string[][])  [unwired: 2 in, 1 out]
        n272 = local write "Spec Default set"(w456) -> ()
        n273 = local write "Condition set"(w490) -> ()
        n274 = local write "Result set 2"(w455) -> ()
        n275 = local write "Resolution"(w489) -> ()
        n276 = call "Variables Data IO.vi"("Write blank data ?(F)"=w459, "Select"=w499, "error in"=w500, "Data In"=w497, "Func_ext"=w501) -> ("error out"=w471:errorcluster, "Func_ext Out"=w469:string)  [unwired: 4 in, 1 out]
        n277 = local write "Result set"(w472) -> ()
        n278 = local write "CMC set"(w479) -> ()
        n279 = local write "Spec set"(w488) -> ()
        n280 = for {
          tunnel: w490 -> [w523] mode=indexing
          tunnel: [w522] -> w503 mode=concatenating
          tunnel: w489 -> [w521] mode=indexing
          tunnel: w488 -> [w520] mode=indexing
          tunnel: [w519] -> w487 mode=concatenating
          tunnel: [w518] -> w486 mode=concatenating
          tunnel: w479 -> [w517] mode=indexing
          tunnel: [w516] -> w475 mode=concatenating
          tunnel: w472 -> [w514] mode=indexing
          tunnel: [w513] -> w467 mode=concatenating
          w515 = enum16{"행", "열", "행,열"}."행" ("조건")
          n281 = call-poly "Remove Empty Array.vi"("조건"=w515, "Data in"=w523) -> ("Data out"=w522:string[][])  [unwired: 8 in, 1 out]
          n282 = call-poly "Remove Empty Array.vi"("조건"=w515, "Data in"=w521) -> ("Data out"=w519:string[][])  [unwired: 8 in, 1 out]
          n283 = call-poly "Remove Empty Array.vi"("조건"=w515, "Data in"=w520) -> ("Data out"=w518:string[][])  [unwired: 8 in, 1 out]
          n284 = call-poly "Remove Empty Array.vi"("조건"=w515, "Data in"=w517) -> ("Data out"=w516:string[][])  [unwired: 8 in, 1 out]
          n285 = call-poly "Remove Empty Array.vi"("조건"=w515, "Data in"=w514) -> ("Data out"=w513:string[][])  [unwired: 8 in, 1 out]
        }
        n286 = call "Variables Data IO.vi"("Select"=Cmd_Var_Data_IO."Result", "error in"=w471, "Data In"=w467, "Func_ext"=w469) -> ("error out"=w470:errorcluster, "Func_ext Out"=w468:string)  [unwired: 5 in, 1 out]
        n287 = call "Variables Data IO.vi"("Write blank data ?(F)"=w459, "Select"=Cmd_Var_Data_IO."CMC", "error in"=w470, "Data In"=w475, "Func_ext"=w468) -> ("error out"=w478:errorcluster, "Func_ext Out"=w477:string)  [unwired: 4 in, 1 out]
        n288 = call "Variables Data IO.vi"("Write blank data ?(F)"=w459, "Select"=Cmd_Var_Data_IO."Spec", "error in"=w478, "Data In"=w486, "Func_ext"=w477) -> ("error out"=w483:errorcluster, "Func_ext Out"=w480:string)  [unwired: 4 in, 1 out]
        n289 = call "Variables Data IO.vi"("Write blank data ?(F)"=w459, "Select"=Cmd_Var_Data_IO."Resolution", "error in"=w483, "Data In"=w487, "Func_ext"=w480) -> ("error out"=w482:errorcluster, "Func_ext Out"=w481:string)  [unwired: 4 in, 1 out]
        n290 = call "Variables Data IO.vi"("Write blank data ?(F)"=w459, "Select"=Cmd_Var_Data_IO."Condition", "error in"=w482, "Data In"=w503, "Func_ext"=w481) -> ("error out"=w504:errorcluster)  [unwired: 4 in, 2 out]
      }
      frame "dut info 초기화" {
        w525 = TRUE ("Write blank data ?(T)")
        w526 = string[][] []
        n291 = property on="dut info" class="MCListbox (엄격한)"(error in=w539, "ItemNames"=w526) -> (error out=w531:errorcluster)  [unwired: 1 in, 1 out]
        n292 = Build Array(w526) -> (w524:string[][][])
        n293 = local write "Condition set"(w524) -> ()
        n294 = local write "Resolution"(w524) -> ()
        n295 = local write "Spec set"(w524) -> ()
        n296 = local write "CMC set"(w524) -> ()
        n297 = local write "Result set"(w524) -> ()
        n298 = local write "Result set 2"(w524) -> ()
        n299 = local write "Spec Default set"(w524) -> ()
        n300 = call "Variables Data IO.vi"("Write blank data ?(F)"=w525, "Select"=Cmd_Var_Data_IO."Condition_Temp", "error in"=w531, "Func_ext"=w529) -> ("error out"=w530:errorcluster, "Func_ext Out"=w528:string)  [unwired: 5 in, 1 out]
        n301 = Build Array(Cmd_Var_Data_IO."STD1" ("Select"), Cmd_Var_Data_IO."CMC" ("Select"), Cmd_Var_Data_IO."Spec" ("Select"), Cmd_Var_Data_IO."Resolution" ("Select"), Cmd_Var_Data_IO."Condition" ("Select")) -> (w532:T3[])
        n302 = for {
          tunnel: w525 -> [w544]
          tunnel: w532 -> [w543] mode=indexing
          tunnel: w528 -> [w542]
          shift-right: [w545] -> w538
          shift-left: w530 -> [w541]
          n303 = call "Variables Data IO.vi"("Write blank data ?(F)"=w544, "Select"=w543, "error in"=w541, "Func_ext"=w542) -> ("error out"=w545:errorcluster)  [unwired: 5 in, 2 out]
        }
      }
      frame "Condition 변경" {
        w550 = TRUE ("Write blank data ?(T)")
        n304 = local read "Condition set"() -> (w577:string[][][])
        n305 = local read "Condition"() -> (w568:string[][])
        n306 = local read "dut info"() -> (w570:i32)
        n307 = Replace Array Subset(array=w577, new element=w568, index (dim 0)=w570) -> (w566:string[][][])  [unwired: 2 in]
        n308 = local write "Condition set"(w566) -> ()
        n309 = call "Variables Data IO.vi"("Select"=Cmd_Var_Data_IO."Spec Temp", "error in"=w576, "Func_ext"=w574) -> ("error out"=w553:errorcluster, "Data Out"=w564:string[][], "Func_ext Out"=w554:string)  [unwired: 6 in]
        n310 = call "Variables Data IO.vi"("Select"=Cmd_Var_Data_IO."CMC Default", "error in"=w553, "Func_ext"=w554) -> ("error out"=w551:errorcluster, "Data Out"=w548:string[][], "Func_ext Out"=w552:string)  [unwired: 6 in]
        n311 = for {
          tunnel: w566 -> [w592] mode=indexing
          tunnel: [w581] -> w561 mode=concatenating
          tunnel: w554 -> [w579]
          tunnel: w564 -> [w582]
          tunnel: [w589] -> w563 mode=indexing
          tunnel: refnum<vi> refnum ("Spec Ref.") -> [w590]
          tunnel: [w589] -> w562 mode=concatenating
          tunnel: w548 -> [w586]
          tunnel: [w585] -> w555 mode=concatenating
          tunnel: [w585] -> w547 mode=indexing
          tunnel: "Resolution" -> [w580] mode=indexing
          tunnel: [w584] -> w546 mode=indexing
          n312 = call-poly "Remove Empty Array.vi"("조건"=enum16{"행", "열", "행,열"}."행", "Data in"=w592) -> ("Data out"=w581:string[][])  [unwired: 8 in, 1 out]
          n313 = call "Get Spec.vi"("NumRows"=u32 0, "Spec in"=w582, "Spec Ref."=w590, "Condition in"=w581, "Resolution in"=w580, "Func_ext"=w579) -> ("Data Out"=w587:string[][], "Spec Out"=w589:string[][], "Func_ext Out"=w588:string, "Spec (Default)"=w584:string[][])  [unwired: 1 in, 1 out]
          n314 = call "Match_CMC.vi"("CMC IN"=w586, "Condition IN"=w587, "Func_ext"=w588) -> ("CMC Out"=w585:string[][])  [unwired: 5 in, 3 out]
        }
        n315 = local write "Spec Default set"(w546) -> ()
        n316 = local write "CMC set"(w547) -> ()
        n317 = Index Array(array=w563, index (dim 0)=w570) -> (element=w569:string[][])  [unwired: 2 in]
        n318 = local write "Spec"(w569) -> ()
        n319 = local write "Spec set"(w563) -> ()
        n320 = call "Variables Data IO.vi"("Write blank data ?(F)"=w550, "Select"=Cmd_Var_Data_IO."Condition", "error in"=w551, "Data In"=w561, "Func_ext"=w552) -> ("error out"=w559:errorcluster, "Func_ext Out"=w560:string)  [unwired: 4 in, 1 out]
        n321 = call "Variables Data IO.vi"("Write blank data ?(F)"=w550, "Select"=Cmd_Var_Data_IO."CMC", "error in"=w559, "Data In"=w555, "Func_ext"=w560) -> ("error out"=w557:errorcluster, "Func_ext Out"=w558:string)  [unwired: 4 in, 1 out]
        n322 = call "Variables Data IO.vi"("Write blank data ?(F)"=w550, "Select"=Cmd_Var_Data_IO."Spec", "error in"=w557, "Data In"=w562, "Func_ext"=w558) -> ("error out"=w573:errorcluster)  [unwired: 4 in, 2 out]
      }
    }
  }
  n323 = Release Queue(queue=w10, error in (no error)=w11) -> (error out=w8:errorcluster)  [unwired: 1 in, 2 out]
  n324 = Merge Errors(w9, w8) -> (→"에러 출력":errorcluster)
